vi "Error Bar Interpolation Write.vi"(4 "error in (no error)":errorcluster, 5 "Value":u8, 6 "Container State":T3, 7 "Display State In":T1) -> (0 "error out":errorcluster, 3 "Display State Out":T1)   [LabVIEW 2017, in "2D Error Bar.xctl"]
uses:
  <vilib>/Math Plots/2D Math Plots/2D Error Bar/2D Error Bar XCtrl/2D Error Bar.xctl
  <vilib>/_xctls/Container State.ctl
  <vilib>/Math Plots/2D Math Plots/2D Error Bar/2D Error Bar XCtrl/State.ctl
  <vilib>/Math Plots/2D Math Plots/2D Error Bar/2D Error Bar/2D Error Bar.lvclass
  e:/builds/penguin/labview/branches/2017/dev/dist/vi.lib/Math Plots/2D Math Plots/2D Plot/2D Plot/2D Plot.lvclass
  <vilib>/Math Plots/2D Math Plots/2D Plot/Action String/2DMathPlot Ctrl Act Queue.ctl
  <vilib>/Math Plots/2D Math Plots/2D Plot/Action String/2DMathPlot Ctrl Act Cluster.ctl
  <vilib>/Math Plots/2D Math Plots/2D Plot/Action String/2DMathPlot State Class.ctl
  <vilib>/Math Plots/2D Math Plots/2D Plot/2D Plot/2D Plot.lvclass
  <vilib>/_xctls/XControlSupport.lvlib
panel:
  # "Replace the Value Control below with a Control of desired type.\nDo not remove this Control or the others from the connector pane.\nDo not change the connector pane pattern.\nThe Value control should always be the third terminal from top on the input side in the connector pane."
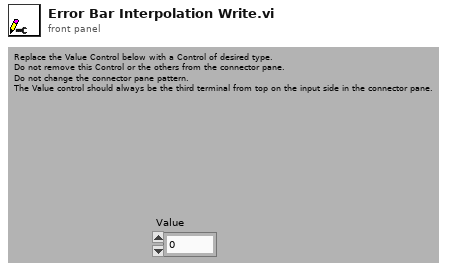
[diagram p1: front panel]
types:
  T1 = typedef "2D Error Bar.xctl/State.ctl" = cluster{"2D Error Bar.lvclass":refnum<class "2D Error Bar.lvclass">, "Control Ref Queue":T2, "Main Frame Color":u32, "Plot Legend Color":u32}
  T2 = typedef "2DMathPlot Ctrl Act Queue.ctl" = refnum<queue>
  T3 = typedef "XControlSupport.lvlib/Container State.ctl" = cluster{"Indicator?":bool, "Run Mode?":bool, " Refnum":refnum<vi>}
  T4 = typedef "2DMathPlot State Class.ctl" = enum16{"Update All (Undo)", "Update General", "Update Appearance", "Update Format", "Update Scale", "Update Marker", "Update Cursor", "None"}
  T5 = typedef "2D Error Bar.lvclass/2D Error Bar Property Array.ctl" = T6[]
  T6 = typedef "2D Error Bar.lvclass/2D Error Bar Property.ctl" = cluster{"Marker Size":dbl, "Marker Line Style":u8, "Marker Line Width":u8, "Marker Color":u32, "Error Bar Interpolation":enum16{"Show Point", "Show Line", "Show Bar"}, "Error Mode":enum16{"Show Y Error", "Show X Error", "Show Both Error"}}
  T7 = typedef "2D Plot.lvclass/Plot Property Array.ctl" = T8[]
  T8 = typedef "2D Plot.lvclass/Plot Property.ctl" = cluster{"Bar Plot Style":u8, "DigitalLineStyle":u8, "TransitionLocation":u8, "Transition Type":u8, "Fill To":i16, "Fill/Pt. Color":u32, "Label Style":u8, "Line Style":u8, "Line Width":u8, "Plot Color":u32, "Plot Interpolation":u8, "Plot Name":string, "Point Style":u8, "Visible?":bool, "XScaleIdx":u32, "YScaleIdx":u32}
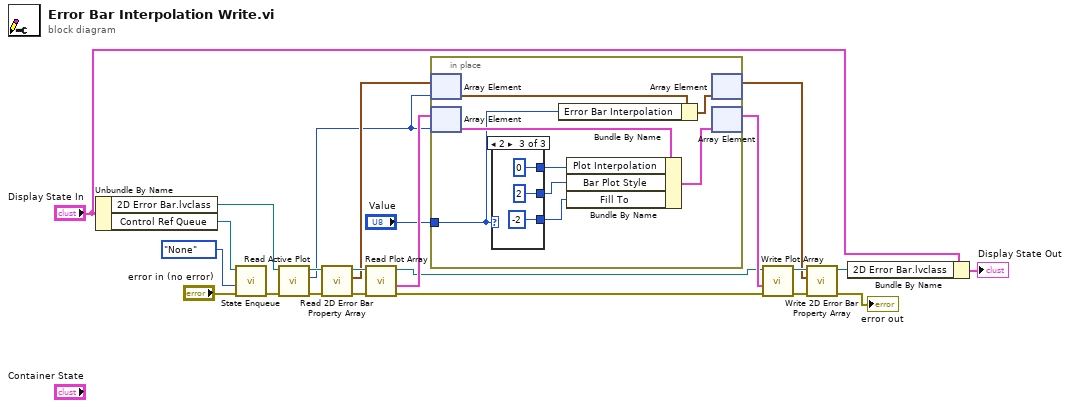
[diagram p0: block diagram]
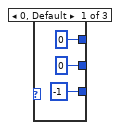
[diagram p2: hidden frame]
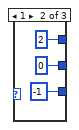
[diagram p3: hidden frame]
diagram:
  n1 = Unbundle By Name("Display State In") -> ("2D Error Bar.lvclass"=w23:refnum<class "2D Error Bar.lvclass">, "Control Ref Queue"=w19:T2)
  n2 = call <vilib>:"State Enqueue.vi"("error in (no error)"="error in (no error)", "Display State Change Class"=2DMathPlot_State_Class."None", "Control Ref Queue"=w19) -> ("error out"=w18:errorcluster)  [unwired: 8 out]
  n3 = call <vilib>:"Read Active Plot.vi"("error in (no error)"=w18, "2D Plot.lvclass in"=w23) -> ("error out"=w13:errorcluster, "Active Plot"=w3:i32, "2D Plot.lvclass out"=w11:refnum<class "2D Error Bar.lvclass">)  [unwired: 7 out]
  n4 = call <vilib>:"Read 2D Error Bar Property Array.vi"("error in (no error)"=w13, "2D Error Bar.lvclass in"=w11) -> ("error out"=w12:errorcluster, "2D Error Bar Property Array"=w4:T5, "2D Error Bar.lvclass out"=w10:refnum<class "2D Error Bar.lvclass">)  [unwired: 7 out]
  n5 = call-dynamic "Read Plot Array.vi"("error in (no error)"=w12, "2D Error Bar.lvclass in"=w10) -> ("error out"=w8:errorcluster, "Plot Property Array"=w22:T7, "2D Error Bar.lvclass out"=w9:refnum<class "2D Error Bar.lvclass">)  [unwired: 7 out]
  n6 = in-place {
    in-place-border: "Value" -> [w24]
    n7 = in-place-array #1(w4, w3) -> (w31:T6)
    n8 = in-place-array #2(w22, w3) -> (w26:T8)
    n9 = case shown="2" w24 {
      tunnel: [u8 0 ("Plot Interpolation") u8 2 ("Plot Interpolation") u8 0 ("Plot Interpolation")] -> w29
      tunnel: [u8 0 ("Plot Interpolation") u8 0 ("Plot Interpolation") u8 2 ("Plot Interpolation")] -> w28
      tunnel: [i16 -1 ("Fill To") i16 -1 ("Fill To") i16 -2 ("Fill To")] -> w27
      frame 0, Default {
      }
      frame 1 {
      }
      frame 2 {
      }
    }
    n10 = Bundle By Name(cluster=w31, "Error Bar Interpolation"=w24) -> (w30:T6)
    n11 = Bundle By Name(cluster=w26, "Plot Interpolation"=w29, "Bar Plot Style"=w28, "Fill To"=w27) -> (w25:T8)
    n12 = in-place-array #1(w30) -> (w2:T5)  [unwired: 1 out]
    n13 = in-place-array #2(w25) -> (w21:T7)  [unwired: 1 out]
  }
  n14 = call-dynamic "Write Plot Array.vi"("error in (no error)"=w8, "Plot Property Array"=w21, "2D Error Bar.lvclass in"=w9) -> ("error out"=w5:errorcluster, "2D Error Bar.lvclass out"=w7:refnum<class "2D Error Bar.lvclass">)  [unwired: 7 out]
  n15 = call <vilib>:"Write 2D Error Bar Property Array.vi"("error in (no error)"=w5, "2D Error Bar Property Array"=w2, "2D Error Bar.lvclass in"=w7) -> ("error out"=→"error out":errorcluster, "2D Error Bar.lvclass out"=w6:refnum<class "2D Error Bar.lvclass">)  [unwired: 1 in, 6 out]
  n16 = Bundle By Name(cluster="Display State In", "2D Error Bar.lvclass"=w6) -> (→"Display State Out":T1)
